vi "daq.io Embedded Machine with Buffering Example.vi"() -> ()   [LabVIEW 2013, in "daqio minimal.lvlib"]
doc: "This interactive example demonstrates how an NI Embedded device can used for continuous monitoring with daq.io. Tags and Events in this example are written on user demand but could also be triggered by monitored values. \n\nTo get started, <b>drag this example onto a Real-Time target in the Project Explorer, enter your credentials in the block diagram</b> and run it interactively. You can also build an Executable and run it upon startup.\n\nClicking \"Create Dashboard\" will generate a dashboard for this device on daq.io.\n\nThe NI System Configuration API is being used to monitor the status of the Embedded device. Please make sure its libraries are installed on the Embedded Device to get the best experience."
uses:
  daqio minimal.lvlib
  _typedefs/update-button.ctl
  _typedefs/trigger-button.ctl
  _typedefs/dashboard-button.ctl
  _typedefs/daqio-Credentials.ctl
  _typedefs/exmpl-states.ctl
  _typedefs/connection_FGV_commands.ctl
  _typedefs/daqio-Buffer-Commands.ctl
  <vilib>/nisyscfg/Close (System).vi
  <resource>/objmgr/nisysapi.rc
  <vilib>/nisyscfg/nisyscfg.lvlib
panel:
  in  "Create Dashboard":T1
  out "Log":string[](array[string])
  in  "Stop":bool
  in  "Fire Event":T2
  in  "Select Event":u16(ring) items=["Safety Hood Status", "Manual Operation", "Shutting Down"]
  out "Time Stamp sent":timestamp
  in  "Event Data":string
  in  "Update Tags":T3
  out "connected":bool
  out "Speed (RPM)":dbl(knob) scale=0.0..2000.0
  out "Temperature Data":dbl(graph)
  out "RAM":dbl(slide) scale=0.0..100.0
  out "CPU":dbl(slide) scale=0.0..100.0
  in  "Setpoint\n(set manually)":dbl(knob) scale=0.0..100.0
  in  "Value 3":string="1234-abc"
  in  "Value 2":string="XYZ 3000 Plus"
  in  "Tag 3":string="Serial Number"
  in  "Tag 2":string="Type"
  in  "Value 1":string="47.615459, -122.323804"
  in  "Tag 1":string="Location"
  in  "error in (no error)":errorcluster
  out "error out":errorcluster
  out "Device Key":string
  out "Device Type Key":string
  out "Dashboard URL - copy and open in your web browser":string
  # "Get your free account at daq.io first: sign up at daq.io."
  # "This Machine"
  # "(autogenerated in this example)"
  # "Please enter your \ncredentials in the \nblock diagram."
  # "Device Tags"
  # "Use device tags to describe \nspecific parameters for each\ndevice. These can include the \nlocation, the serial number or\nother machine or location-\nspecific information. These\nfields are fully user-defined."
  # "Device Events"
  # "Use device events to signal\nany local event to daq.io. These\ncould include mechanical events\n(e.g. \"safety latch released\") or \nany change on the device that\nneeds to be tracked."
  # "Device Live Data Channels"
  # "Use device channels to transfer\ntime series data. All channels \nof the device will be visible in \nthe online data viewer. You \ncan build your own dashboard \nin the webbrowser and link it\nto exisiting channels. Clicking\n\"Create Dashboard\" will\ngenerate a dashboard \nfor this example."
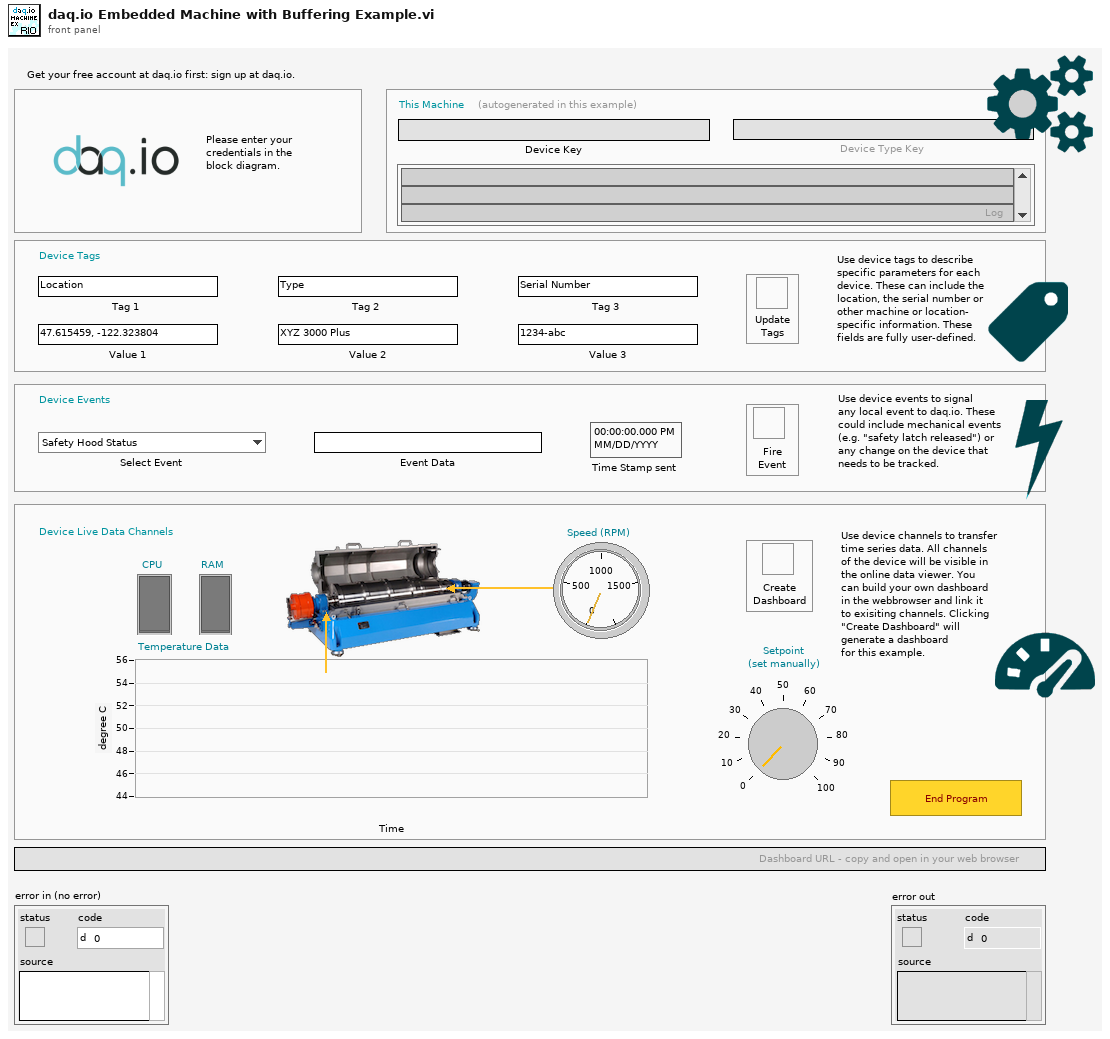
[diagram p1: front panel]
types:
  T1 = typedef "daqio minimal.lvlib/dashboard-button.ctl" = bool
  T2 = typedef "daqio minimal.lvlib/trigger-button.ctl" = bool
  T3 = typedef "daqio minimal.lvlib/update-button.ctl" = bool
  T4 = typedef "daqio minimal.lvlib/exmpl-states.ctl" = enum16{"idle", "time series", "fire events", "update tags", "end program", "create dashboard"}
  T5 = typedef "daqio minimal.lvlib/daqio-Credentials.ctl" = cluster{"User Name":string, "Password":string}
  T6 = typedef "daqio minimal.lvlib/daqio-Type.ctl" = cluster{"daq.io ref":T7, "daq.io API Base":string, "Device Type Key":string, "Device Key":string, "Account ID":string, "online":bool}
  T7 = typedef "LabVIEWHTTPClient.lvlib/ClientHandle.ctl" = refnum<k1>
  T8 = typedef "daqio minimal.lvlib/connection_FGV_commands.ctl" = enum16{"Set Type", "Set Buffer", "Get"}
  T9 = typedef "daqio minimal.lvlib/daqio-Buffer-Commands.ctl" = enum16{"Add to Buffer", "Post from Buffer", "Clear Buffer", "Init"}
  T10 = enum8{"Enabled", "Disabled", "Disabled and Grayed Out"}
  T11 = enum16{"Reconnect success", "Reconnect failed", "Connected"}
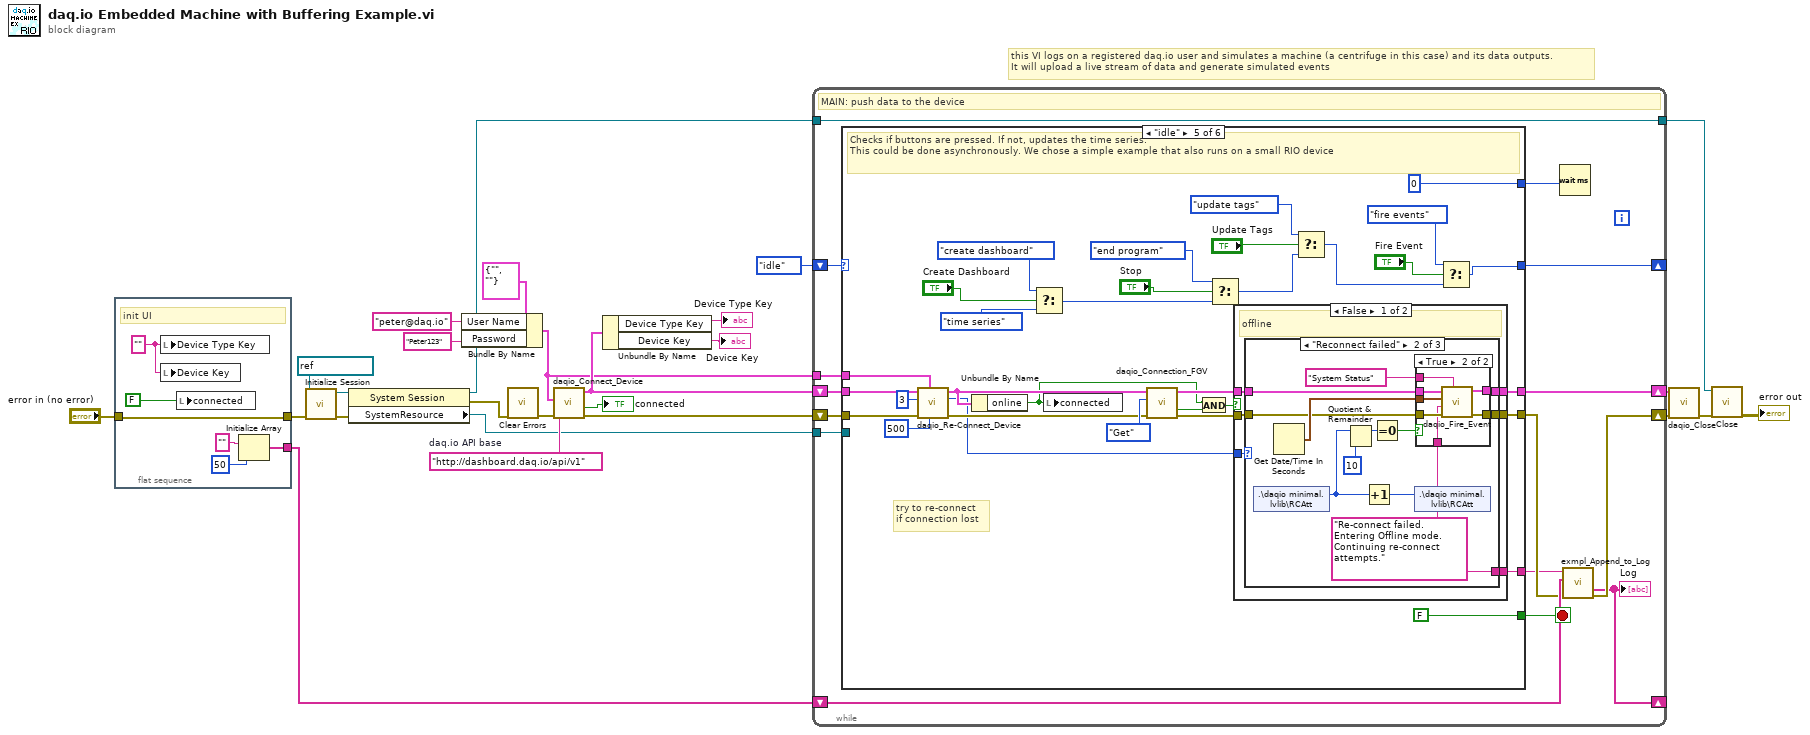
[diagram p0: block diagram]
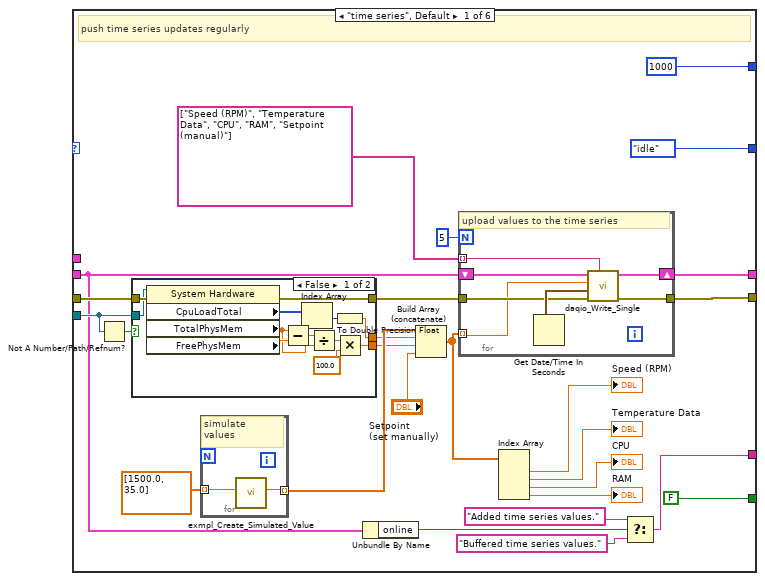
[diagram p2: hidden frame]
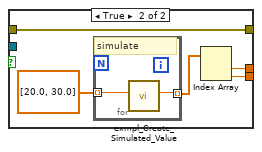
[diagram p3: hidden frame]
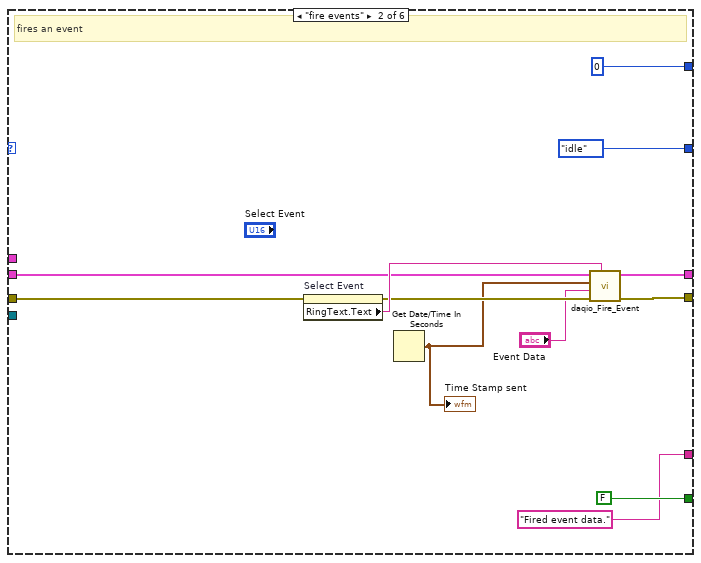
[diagram p4: hidden frame]
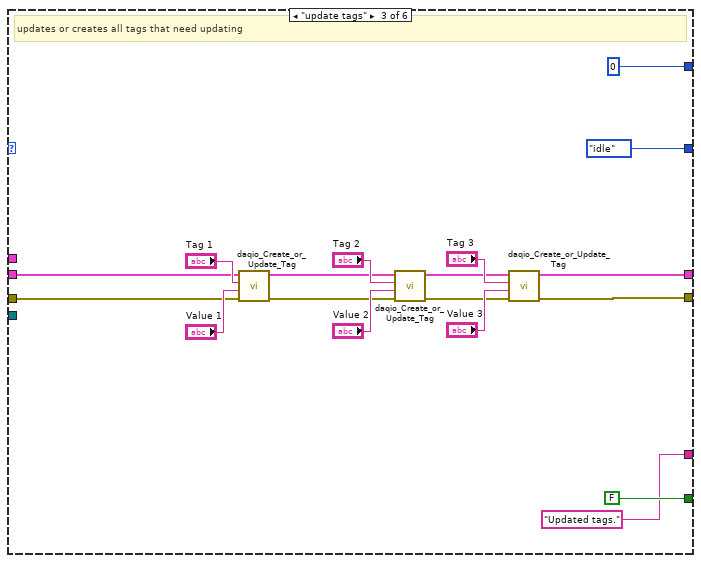
[diagram p5: hidden frame]
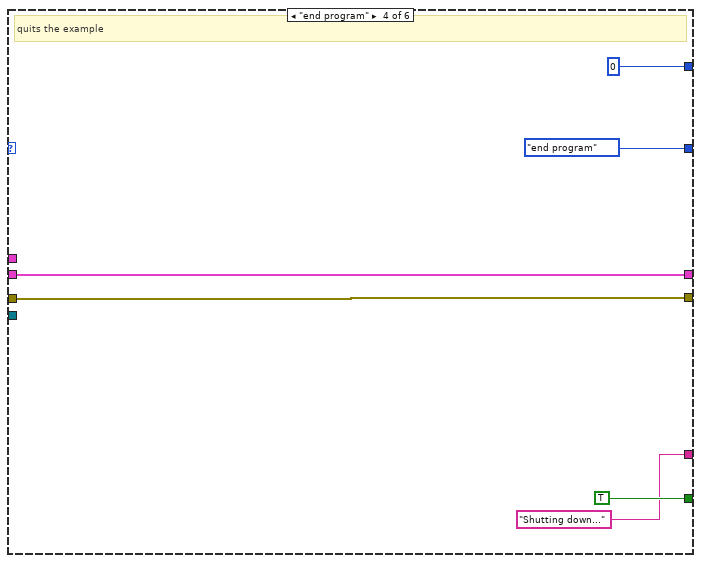
[diagram p6: hidden frame]
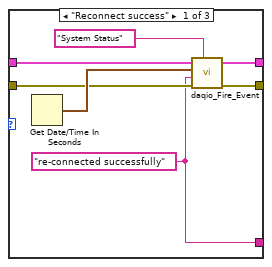
[diagram p7: hidden frame]
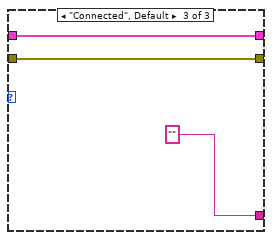
[diagram p9: hidden frame]
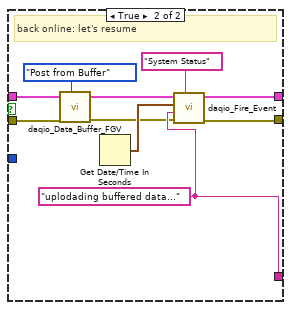
[diagram p10: hidden frame]
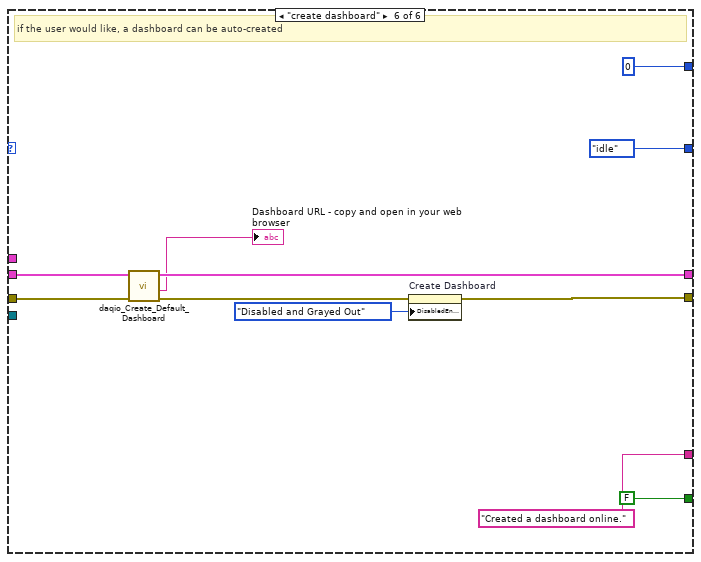
[diagram p11: hidden frame]
diagram:
  w22 = "http://dashboard.daq.io/api/v1"  # daq.io API base
  # "this VI logs on a registered daq.io user and simulates a machine (a centrifuge in this case) and its data outputs. \nIt will upload a live stream of data and generate simulated events"
  n1 = flat-sequence {
    tunnel: [w28] -> w17
    tunnel: "error in (no error)" -> [w28]
    tunnel: [w27] -> w4
    frame #0 {
      w32 = "" ("log")
      # "init UI"
      n2 = local write "Device Type Key"(w32) -> ()
      n3 = local write "Device Key"(w32) -> ()
      n4 = local write "connected"(FALSE ("connected to daq.io")) -> ()
      n5 = Initialize Array("" ("log"), 50 ("dimension size")) -> (w27:string[])
    }
  }
  n6 = call <vilib>:"Initialize Session.vi"("error in (no error)"=w17, "target (localhost)"=refnum<k21> "localhost" ("Embedded Target (self)")) -> ("error out"=w11:errorcluster, "session out"=w9:refnum<k21>)  [unwired: 8 in]
  n7 = property class="System Session"(reference=w9, error in=w11) -> (reference out=w8:refnum<k21>, error out=w10:errorcluster, "SystemResource"=w12:refnum<k20>)
  n8 = Bundle By Name(cluster=T5 {"User Name"="", "Password"=""} ("daq.io Credentials"), "User Name"="peter@daq.io", "Password"="Peter123") -> (w1:T5)
  n9 = call <vilib>:"Clear Errors.vi"("error in (no error)"=w10) -> ("error out"=w18:errorcluster)  [unwired: 6 in]
  n10 = call "daqio_Connect_Device.vi"("daq.io API base"=w22, "error in (no error)"=w18, "Credentials"=w1) -> ("error out"=w2:errorcluster, "connected successfully?"=→"connected":bool, "daq.io type out"=w3:T6)  [unwired: 5 in, 1 out]
  n11 = Unbundle By Name(w3) -> ("Device Type Key"=→"Device Type Key":string, "Device Key"=→"Device Key":string)
  n12 = while {
    shift-right: [w38] -> w26
    shift-left: w2 -> [w35]
    shift-right: [w47] -> w24
    shift-left: w3 -> [w36]
    shift-right: [w45] -> _
    shift-left: exmpl-states."idle" -> [w46]
    tunnel: w12 -> [w42]
    tunnel: [w41] -> w14
    tunnel: w8 -> [w41]
    shift-right: [w37] -> _
    shift-left: w4 -> [w40]
    tunnel: w1 -> [w34]
    stop <- w44 stop-if-true
    # "MAIN: push data to the device"
    n13 = case shown="\"idle\"" w46 {
      tunnel: w36 -> [w52 w110 w121 w135 w148 w223]
      tunnel: w35 -> [w59 w109 w120 w134 w147 w222]
      tunnel: [w66 w107 w118 w135 w151 w221] -> w47
      tunnel: [w65 w108 w119 w134 w150 w217] -> w39
      tunnel: [exmpl-states."idle" exmpl-states."idle" exmpl-states."idle" exmpl-states."end program" w166 exmpl-states."idle"] -> w45
      tunnel: [FALSE FALSE FALSE TRUE FALSE FALSE] -> w44
      tunnel: [u32 1000 ("milliseconds to wait") u32 0 ("milliseconds to wait") u32 0 ("milliseconds to wait") u32 0 ("milliseconds to wait") u32 0 ("milliseconds to wait") u32 0 ("milliseconds to wait")] -> w43
      tunnel: [w48 "Fired event data." ("log") "Updated tags." ("log") "Shutting down..." ("log") w139 "Created a dashboard online." ("log")] -> w33
      tunnel: w42 -> [w56 _ _ _ _ _]
      tunnel: w34 -> [_ _ _ _ w149 _]
      frame "time series", Default {
        # "push time series updates regularly"
        n14 = Not A Number/Path/Refnum?(number/path/refnum=w56) -> (NaN/Path/Refnum?=w55:bool)
        n15 = case shown="False" w55 {
          tunnel: w59 -> [w85 w86]
          tunnel: w56 -> [w84 _]
          tunnel: [w83 w86] -> w58
          tunnel: [w79 w87] -> w57
          tunnel: [w77 w88] -> w54
          frame False {
            n16 = property class="System Hardware"(reference=w84, error in=w85) -> (error out=w83:errorcluster, "CpuLoadTotal"=w82:u32[], "TotalPhysMem"=w74:dbl, "FreePhysMem"=w75:dbl)  [unwired: 1 out]
            n17 = Subtract(x=w74, y=w75) -> (x-y=w76:dbl)
            n18 = Index Array(array=w82) -> (element=w78:u32)  [unwired: 1 in]
            n19 = Divide(x=w76, y=w74) -> (x/y=w81:dbl)
            n20 = To Double Precision Float(number=w78) -> (double precision float=w77:dbl)
            n21 = Multiply(x=w81, y=100.0) -> (x*y=w79:dbl)
          }
          frame True {
            n22 = for {
              tunnel: [w92] -> w89 mode=indexing
              tunnel: dbl[] [20.0, 30.0] -> [w91] mode=indexing
              # "simulate"
              n23 = call "exmpl_Create_Simulated_Value.vi"("offset"=w91) -> ("Numeric"=w92:dbl)  [unwired: 9 in, 1 out]
            }
            n24 = Index Array(array=w89) -> (element #1=w88:dbl, element #2=w87:dbl)  [unwired: 2 in]
          }
        }
        n25 = for {
          tunnel: [w101] -> w72 mode=indexing
          tunnel: dbl[] [1500.0, 35.0] -> [w100] mode=indexing
          # "simulate\nvalues"
          n26 = call "exmpl_Create_Simulated_Value.vi"("offset"=w100) -> ("Numeric"=w101:dbl)  [unwired: 9 in, 1 out]
        }
        n27 = Unbundle By Name(w52) -> ("online"=w51:bool)
        n28 = Build Array (concatenate)(w72, w54, w57, "Setpoint\n(set manually)") -> (w53:dbl[])
        n29 = for {
          N: 5 -> [_]
          tunnel: w53 -> [w97] mode=indexing
          shift-right: [w95] -> w66
          shift-left: w52 -> [w96]
          tunnel: string[] ["Speed (RPM)", "Temperature Data", "CPU", "RAM", "Setpoint (manual)"] -> [w93] mode=indexing
          tunnel: w58 -> [w98]
          tunnel: [w94] -> w65
          # "upload values to the time series"
          n30 = Get Date/Time In Seconds() -> (seconds since 1Jan1904=w99:timestamp)
          n31 = call "daqio_Write_Single.vi"("daq.io Device Channel"=w93, "error in (no error)"=w98, "timestamp"=w99, "value"=w97, "daq.io type in"=w96) -> ("error out"=w94:errorcluster, "daq.io type out"=w95:T6)  [unwired: 5 in]
        }
        n32 = Index Array(array=w53) -> (element #1=→"Speed (RPM)":dbl, element #2=→"Temperature Data":dbl, element #3=→"CPU":dbl, element #4=→"RAM":dbl)  [unwired: 4 in]
        n33 = Select(t="Added time series values." ("log"), s=w51, f="Buffered time series values." ("log")) -> (s? t:f=w48:string)
      }
      frame "fire events" {
        # "fires an event"
        n34 = property on="Select Event" class="Ring (strict)"(error in=w109) -> (error out=w112:errorcluster, "RingText.Text"=w113:string)  [unwired: 1 in, 1 out]
        n35 = Get Date/Time In Seconds() -> (seconds since 1Jan1904=w102:timestamp)
        "Time Stamp sent" <- w102
        n36 = call "daqio_Fire_Event.vi"("Event Key"=w113, "error in (no error)"=w112, "Event Value"="Event Data", "Event Date and Time"=w102, "daq.io type in"=w110) -> ("error out"=w108:errorcluster, "daq.io type out"=w107:T6)  [unwired: 5 in]
      }
      frame "update tags" {
        # "updates or creates all tags that need updating"
        n37 = call "daqio_Create_or_Update_Tag.vi"("error in (no error)"=w120, "Tag Value"="Value 1", "Tag Key"="Tag 1", "daq.io type in"=w121) -> ("error out"=w125:errorcluster, "daq.io type out"=w122:T6)  [unwired: 5 in, 1 out]
        n38 = call "daqio_Create_or_Update_Tag.vi"("error in (no error)"=w125, "Tag Value"="Value 2", "Tag Key"="Tag 2", "daq.io type in"=w122) -> ("error out"=w124:errorcluster, "daq.io type out"=w123:T6)  [unwired: 5 in, 1 out]
        n39 = call "daqio_Create_or_Update_Tag.vi"("error in (no error)"=w124, "Tag Value"="Value 3", "Tag Key"="Tag 3", "daq.io type in"=w123) -> ("error out"=w119:errorcluster, "daq.io type out"=w118:T6)  [unwired: 5 in, 1 out]
      }
      frame "end program" {
        # "quits the example"
      }
      frame "idle" {
        # "try to re-connect\nif connection lost"
        # "Checks if buttons are pressed. If not, updates the time series. \nThis could be done asynchronously. We chose a simple example that also runs on a small RIO device"
        n40 = call "daqio_Re-Connect_Device.vi"("re-connect timeouts"=u32 500, "Credentials"=w149, "error in (no error)"=w147, "re-connect attempts"=3, "daq.io type in"=w148) -> ("error out"=w146:errorcluster, "status"=w144:T11, "daq.io type out"=w145:T6)  [unwired: 4 in]
        n41 = Unbundle By Name(w145) -> ("online"=w138:bool)
        n42 = Select(t=exmpl-states."create dashboard", s="Create Dashboard", f=exmpl-states."time series") -> (s? t:f=w155:T4)
        n43 = local write "connected"(w138) -> ()
        n44 = call "daqio_Connection_FGV.vi"("error in (no error)"=w146, "Enum"=connection_FGV_commands."Get", "daq.io type in"=w145) -> ("error out"=w152:errorcluster, "Buffered Data exists?"=w142:bool, "daq.io type out"=w153:T6)  [unwired: 6 in]
        n45 = And(x=w138, y=w142) -> (x .and. y?=w143:bool)
        n46 = Select(t=exmpl-states."end program", s="Stop", f=w155) -> (s? t:f=w160:T4)
        n47 = case shown="False" w143 {
          tunnel: w153 -> [w170 w215]
          tunnel: w152 -> [w171 w214]
          tunnel: [w175 w212] -> w139
          tunnel: [w173 w208] -> w151
          tunnel: [w172 w207] -> w150
          tunnel: w144 -> [w174 _]
          frame False {
            # "offline"
            n48 = case shown="\"Reconnect failed\"" w174 {
              tunnel: [w176 w188 ""] -> w175
              tunnel: [w180 w189 w205] -> w173
              tunnel: [w179 w190 w204] -> w172
              tunnel: w171 -> [w178 w192 w204]
              tunnel: w170 -> [w177 w191 w205]
              frame "Reconnect success" {
                w176 = "re-connected successfully"
                n49 = Get Date/Time In Seconds() -> (seconds since 1Jan1904=w182:timestamp)
                n50 = call "daqio_Fire_Event.vi"("Event Key"="System Status", "error in (no error)"=w178, "Event Value"=w176, "Event Date and Time"=w182, "daq.io type in"=w177) -> ("error out"=w179:errorcluster, "daq.io type out"=w180:T6)  [unwired: 5 in]
              }
              frame "Reconnect failed" {
                w188 = "Re-connect failed. Entering Offline mode. Continuing re-connect attempts."
                n51 = shared-variable ".\\daqio minimal.lvlib\\RCAtt"() -> (w184:i32)  [unwired: 1 in, 1 out]
                n52 = Get Date/Time In Seconds() -> (seconds since 1Jan1904=w194:timestamp)
                n53 = Quotient & Remainder(x=w184, y=10) -> (x-y*floor(x/y)=w187:i32)  [unwired: 1 out]
                n54 = Increment(x=w184) -> (x+1=w183:i32)
                n55 = Equal To 0?(x=w187) -> (x = 0?=w186:bool)
                n56 = shared-variable ".\\daqio minimal.lvlib\\RCAtt"(w183) -> ()  [unwired: 1 in, 1 out]
                n57 = case shown="True" w186 {
                  tunnel: w194 -> [_ w203]
                  tunnel: "System Status" ("Event Key") -> [_ w202]
                  tunnel: w192 -> [w195 w201]
                  tunnel: w191 -> [w196 w200]
                  tunnel: [w195 w199] -> w190
                  tunnel: [w196 w198] -> w189
                  tunnel: w188 -> [_ w197]
                  frame False {
                  }
                  frame True {
                    n58 = call "daqio_Fire_Event.vi"("Event Key"=w202, "error in (no error)"=w201, "Event Value"=w197, "Event Date and Time"=w203, "daq.io type in"=w200) -> ("error out"=w199:errorcluster, "daq.io type out"=w198:T6)  [unwired: 5 in]
                  }
                }
              }
              frame "Connected", Default {
              }
            }
          }
          frame True {
            w212 = "uplodading buffered data..."
            # "back online: let's resume"
            n59 = call "daqio_Data_Buffer_FGV.vi"("Buffer Command"=daqio-Buffer-Commands."Post from Buffer", "error in (no error)"=w214, "daq.io type in"=w215) -> ("error out"=w210:errorcluster, "daq.io type out"=w211:T6)  [unwired: 7 in]
            n60 = Get Date/Time In Seconds() -> (seconds since 1Jan1904=w213:timestamp)
            n61 = call "daqio_Fire_Event.vi"("Event Key"="System Status", "error in (no error)"=w210, "Event Value"=w212, "Event Date and Time"=w213, "daq.io type in"=w211) -> ("error out"=w207:errorcluster, "daq.io type out"=w208:T6)  [unwired: 5 in]
          }
        }
        n62 = Select(t=exmpl-states."update tags", s="Update Tags", f=w160) -> (s? t:f=w167:T4)
        n63 = Select(t=exmpl-states."fire events", s="Fire Event", f=w167) -> (s? t:f=w166:T4)
      }
      frame "create dashboard" {
        # "if the user would like, a dashboard can be auto-created"
        n64 = call "daqio_Create_Default_Dashboard.vi"("error in (no error)"=w222, "daq.io type in"=w223) -> ("error out"=w218:errorcluster, "Dashboard URL"=→"Dashboard URL - copy and open in your web browser":string, "daq.io type out"=w221:T6)  [unwired: 6 in, 1 out]
        n65 = property on="Create Dashboard" class="Bool"(error in=w218, "DisabledEnum"=T10."Disabled and Grayed Out" ("Disabled")) -> (error out=w217:errorcluster)  [unwired: 1 in, 1 out]
      }
    }
    n66 = Wait (ms)(milliseconds to wait=w43) -> ()  [unwired: 1 out]
    n67 = call "exmpl_Append_to_Log.vi"("error in (no error)"=w39, "Log Array in"=w40, "Log Message"=w33) -> ("error out"=w38:errorcluster, "Log Array out"=w37:string[])  [unwired: 7 in]
    "Log" <- w37
  }
  n68 = call "daqio_Close.vi"("error in (no error)"=w26, "daq.io type"=w24) -> ("error out"=w16:errorcluster)  [unwired: 9 in]
  n69 = call-poly <vilib>:"Close.vi"("error in (no error)"=w16, "session in"=w14) -> ("error out"=→"error out":errorcluster)  [unwired: 9 in]
